vi "Alarms Read.vi"(8 "Error In":errorcluster, 10 "InterfaceData":T1 {"GenEast"."TotalFuel(L)" format="%.2f"; "GenEast"."FuelRate(L/H)" format="%.2f"; "GenEast"."ApparentPower(VA)" format="%.2f"; "GenEast"."BattVoltage(V)" format="%.2f"; "GenEast"."Freq(Hz)" format="%.2f"; "GenEast"."RunHours(hr)" format="%.2f"; "GenEast"."PowerFactor" format="%.2f"; "GenEast"."ReactivePower(VAR)" format="%.2f"; "GenEast"."ActivePower(W)" format="%.2f"; "GenWest"."TotalFuel(L)" format="%.2f"; "GenWest"."FuelRate(L/H)" format="%.2f"; "GenWest"."ApparentPower(VA)" format="%.2f"; "GenWest"."BattVoltage(V)" format="%.2f"; "GenWest"."Freq(Hz)" format="%.2f"; "GenWest"."RunHours(hr)" format="%.2f"; "GenWest"."PowerFactor" format="%.2f"; "GenWest"."ReactivePower(VAR)" format="%.2f"; "GenWest"."ActivePower(W)" format="%.2f"; "Converter Alarms 2" format="%016b"; "Converter Faults 2" format="%016b"; "Controller Faults" format="%016b"; "System Status" format="%016b"; "Converter Alarms 1" format="%016b"; "Converter Faults 1" format="%016b"; "Solar Faults" format="%016b"; "ES Rack 10 Alarms" format="%016b"; "ES Rack 9 Alarms" format="%016b"; "ES Rack 8 Alarms" format="%016b"; "ES Rack 7 Alarms" format="%016b"; "ES Rack 6 Alarms" format="%016b"; "ES Rack 5 Alarms" format="%016b"; "ES Rack 4 Alarms" format="%016b"; "ES Rack 3 Alarms" format="%016b"; "ES Rack 2 Alarms" format="%016b"; "ES Rack 1 Alarms" format="%016b"; "ES System Alarms" format="%016b"; "System Faults" format="%016b"; "ES Rack 10 Faults" format="%016b"; "ES Rack 9 Faults" format="%016b"; "ES Rack 8 Faults" format="%016b"; "ES Rack 7  Faults" format="%016b"; "ES Rack 6 Faults" format="%016b"; "ES Rack 5 Faults" format="%016b"; "ES Rack 4 Faults" format="%016b"; "ES Rack 3 Faults" format="%016b"; "ES Rack 2 Faults" format="%016b"; "ES Rack 1 Faults" format="%016b"; "ES System Faults" format="%016b"}, 11 "Alarms Data In":T3) -> (0 "Error Out":errorcluster, 3 "Alarms Data Out":T3)   [LabVIEW 2014]
uses:
  Controls/Alarms Data.ctl
  Controls/Interface Data.ctl
  Controls/Gen Data.ctl
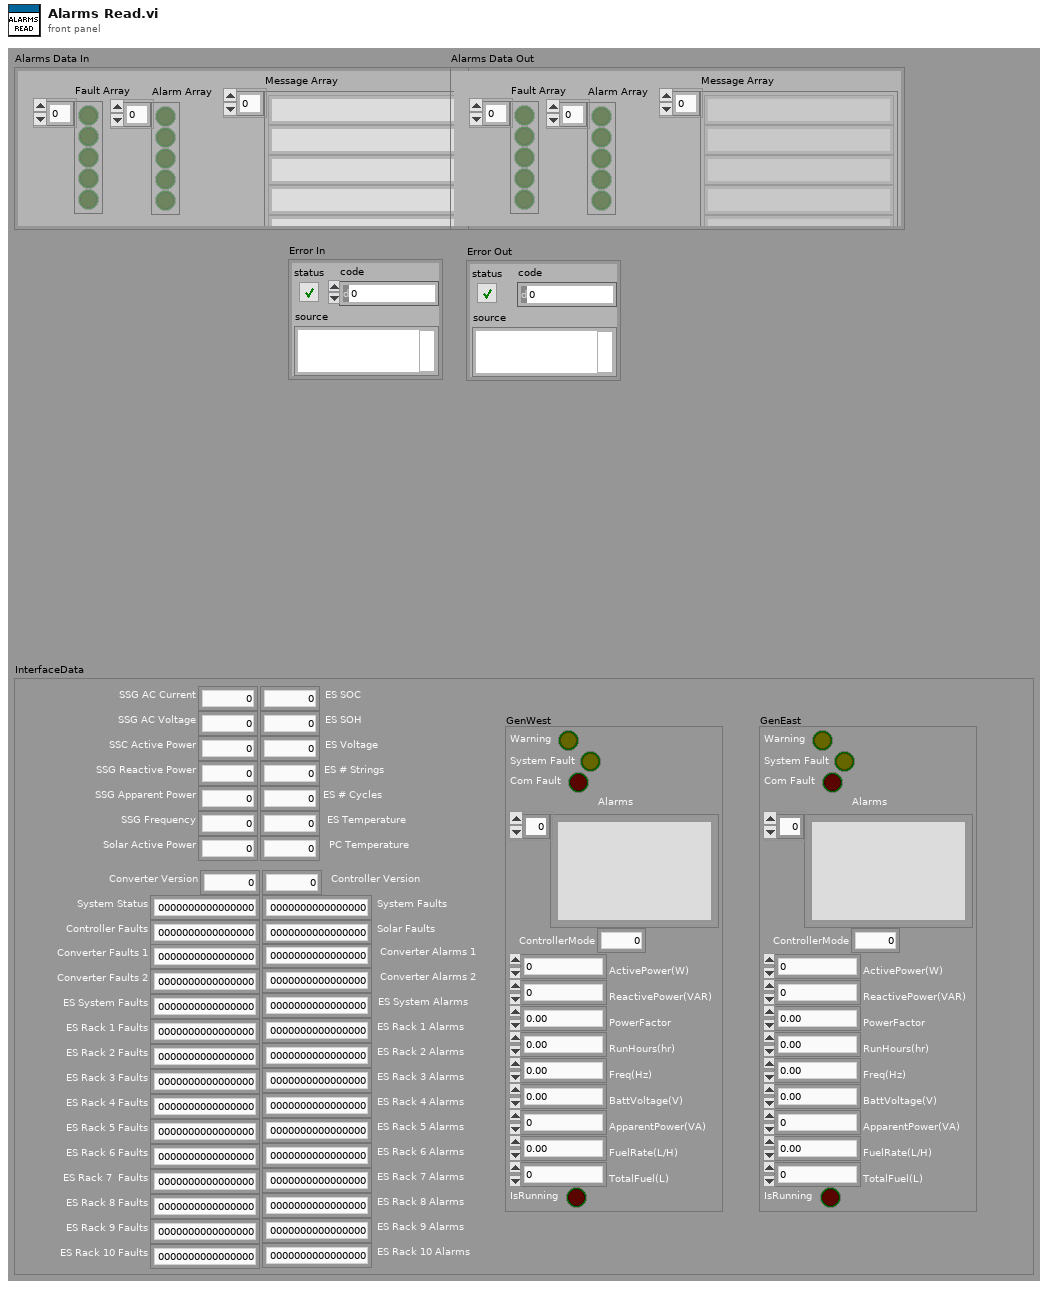
[diagram p1: front panel]
types:
  T1 = typedef "Interface Data.ctl" = cluster{"SSG AC Current":i16, "SSG AC Voltage":i16, "SSC Active Power":i16, "SSG Reactive Power":i16, "SSG Apparent Power":i16, "SSG Frequency":i16, "ES SOC":i16, "ES SOH":i16, "ES Voltage":i16, "ES # Strings":i16, "ES # Cycles":i16, "ES Temperature":i16, "PC Temperature":i16, "Solar Active Power":i16, "Converter Version":i16, "Controller Version":i16, "System Status":i16, "System Faults":i16, "Controller Faults":i16, "ES System Faults":i16, "ES System Alarms":i16, "Converter Faults 1":i16, "Converter Faults 2":i16, "Converter Alarms 1":i16, "Converter Alarms 2":i16, "Solar Faults":i16, "ES Rack 1 Faults":i16, "ES Rack 2 Faults":i16, "ES Rack 3 Faults":i16, "ES Rack 4 Faults":i16, "ES Rack 5 Faults":i16, "ES Rack 6 Faults":i16, "ES Rack 7  Faults":i16, "ES Rack 8 Faults":i16, "ES Rack 9 Faults":i16, "ES Rack 10 Faults":i16, "ES Rack 1 Alarms":i16, "ES Rack 2 Alarms":i16, "ES Rack 3 Alarms":i16, "ES Rack 4 Alarms":i16, "ES Rack 5 Alarms":i16, "ES Rack 6 Alarms":i16, "ES Rack 7 Alarms":i16, "ES Rack 8 Alarms":i16, "ES Rack 9 Alarms":i16, "ES Rack 10 Alarms":i16, "GenWest":T2, "GenEast":T2}
  T2 = typedef "Gen Data.ctl" = cluster{"Warning":bool, "System Fault":bool, "Com Fault":bool, "Alarms":string[], "ControllerMode":u16, "ActivePower(W)":i32, "ReactivePower(VAR)":i32, "PowerFactor":dbl, "RunHours(hr)":dbl, "Freq(Hz)":dbl, "BattVoltage(V)":dbl, "ApparentPower(VA)":i32, "FuelRate(L/H)":dbl, "TotalFuel(L)":u32, "IsRunning":bool}
  T3 = typedef "Alarms Data.ctl" = cluster{"Message Array":string[], "Fault Array":bool[], "Alarm Array":bool[]}
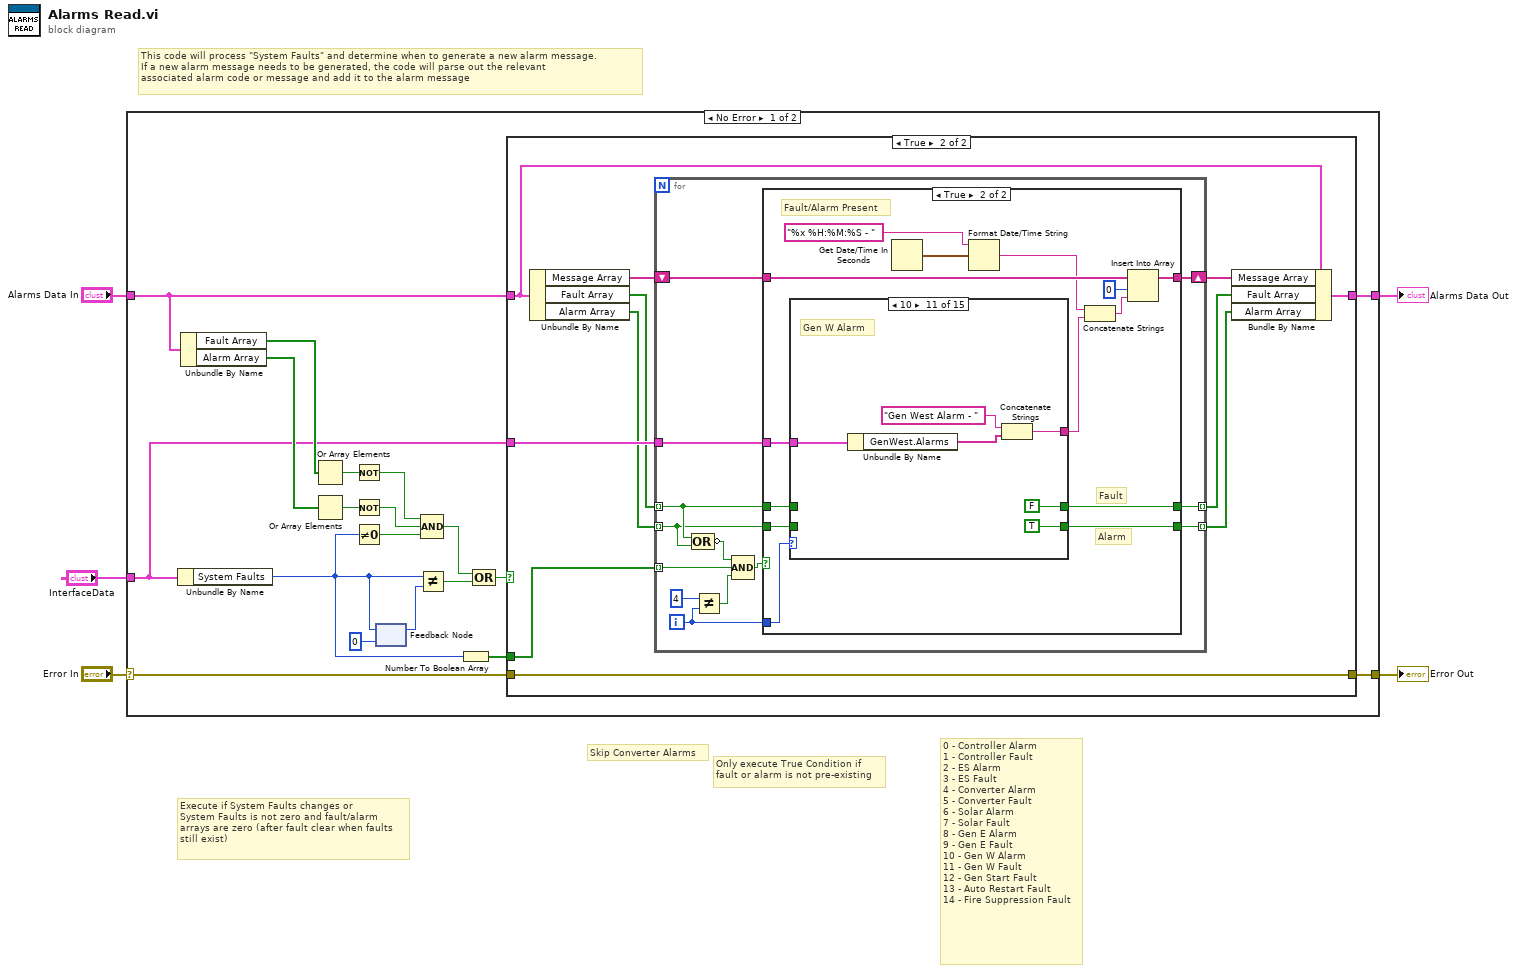
[diagram p0: block diagram]
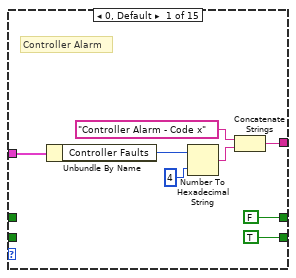
[diagram p4: hidden frame]
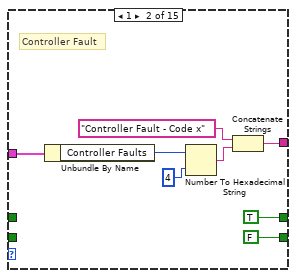
[diagram p5: hidden frame]
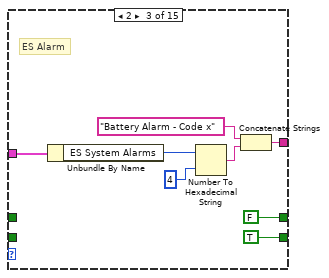
[diagram p6: hidden frame]
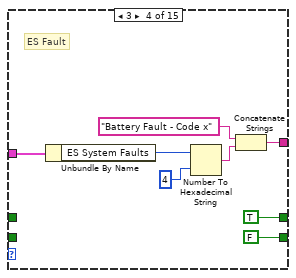
[diagram p7: hidden frame]
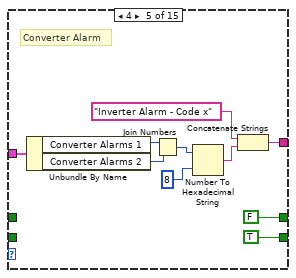
[diagram p8: hidden frame]
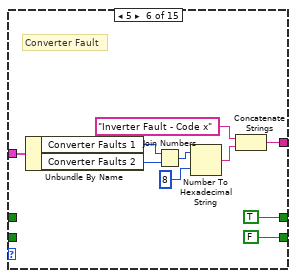
[diagram p9: hidden frame]
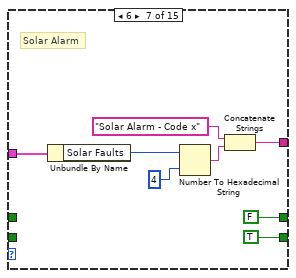
[diagram p10: hidden frame]
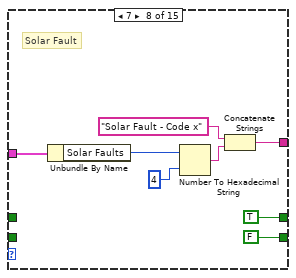
[diagram p11: hidden frame]
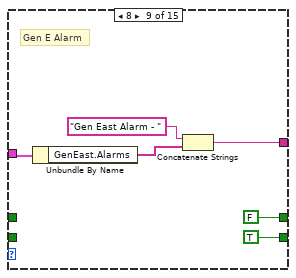
[diagram p12: hidden frame]
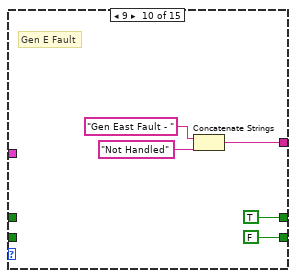
[diagram p13: hidden frame]
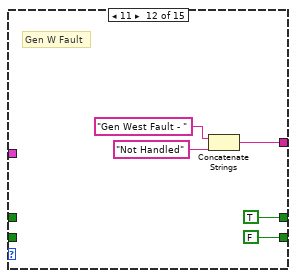
[diagram p14: hidden frame]
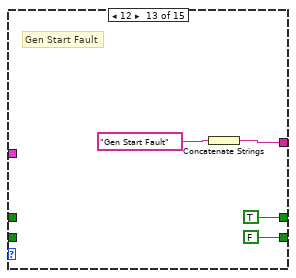
[diagram p15: hidden frame]
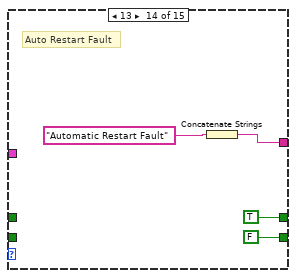
[diagram p16: hidden frame]
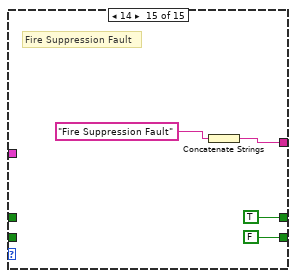
[diagram p17: hidden frame]
diagram:
  # "Skip Converter Alarms"
  # "This code will process \"System Faults\" and determine when to generate a new alarm message.  \nIf a new alarm message needs to be generated, the code will parse out the relevant \nassociated alarm code or message and add it to the alarm message"
  # "Execute if System Faults changes or \nSystem Faults is not zero and fault/alarm\narrays are zero (after fault clear when faults \nstill exist)"
  # "Only execute True Condition if \nfault or alarm is not pre-existing"
  # "0 - Controller Alarm\n1 - Controller Fault\n2 - ES Alarm\n3 - ES Fault\n4 - Converter Alarm\n5 - Converter Fault\n6 - Solar Alarm\n7 - Solar Fault\n8 - Gen E Alarm\n9 - Gen E Fault\n10 - Gen W Alarm\n11 - Gen W Fault\n12 - Gen Start Fault\n13 - Auto Restart Fault\n14 - Fire Suppression Fault"
  n1 = case shown="No Error" "Error In" {
    selector: "Error In" -> [w24 w171]
    tunnel: [w23 w171] -> w4
    tunnel: "Alarms Data In" -> [w17 w170]
    tunnel: [w20 w170] -> w2
    tunnel: "InterfaceData" -> [w9 _]
    frame No Error {
      n2 = Unbundle By Name(w9) -> ("System Faults"=w6:i16)
      n3 = Unbundle By Name(w17) -> ("Fault Array"=w15:bool[], "Alarm Array"=w14:bool[])
      n4 = Or Array Elements(Boolean array=w15) -> (logical OR=w8:bool)
      n5 = Or Array Elements(Boolean array=w14) -> (logical OR=w7:bool)
      n6 = Not(x=w8) -> (.not. x?=w11:bool)
      n7 = Not(x=w7) -> (.not. x?=w12:bool)
      n8 = Not Equal To 0?(x=w6) -> (x != 0?=w16:bool)
      n9 = feedback-in #1(w6) -> ()
      n10 = feedback #1(i16 0 ("System Faults (30052)")) -> (w21:i16)
      n11 = Not Equal?(x=w6, y=w21) -> (x != y?=w19:bool)
      n12 = Compound Arithmetic op=AND(w11, w12, w16) -> (w13:bool)
      n13 = Number To Boolean Array(number=w6) -> (Boolean array=w10:bool[])
      n14 = Compound Arithmetic op=OR(w13, w19) -> (w18:bool)
      n15 = case shown="True" w18 {
        tunnel: w24 -> [w25 w37]
        tunnel: [w25 w37] -> w23
        tunnel: w17 -> [w26 w29]
        tunnel: [w26 w36] -> w20
        tunnel: w10 -> [_ w35]
        tunnel: w9 -> [_ w34]
        frame False {
        }
        frame True {
          n16 = Unbundle By Name(w29) -> ("Message Array"=w30:string[], "Fault Array"=w33:bool[], "Alarm Array"=w32:bool[])
          n17 = for {
            tunnel: w35 -> [w45] mode=indexing
            tunnel: w34 -> [w50]
            tunnel: w33 -> [w43] mode=indexing
            tunnel: w32 -> [w42] mode=indexing
            shift-right: [w48] -> w31
            shift-left: w30 -> [w49]
            tunnel: [w47] -> w28 mode=indexing
            tunnel: [w46] -> w27 mode=indexing
            i -> [w40]
            n18 = Compound Arithmetic op=OR(w43, w42) -> (invert w41:bool)
            n19 = Not Equal?(x=4, y=w40) -> (x != y?=w39:bool)
            n20 = Compound Arithmetic op=AND(w41, w45, w39) -> (w44:bool)
            n21 = case shown="True" w44 {
              tunnel: w40 -> [_ w67]
              tunnel: w50 -> [_ w66]
              tunnel: w49 -> [w53 w65]
              tunnel: [w53 w63] -> w48
              tunnel: w43 -> [w52 w62]
              tunnel: [w52 w59] -> w47
              tunnel: w42 -> [w51 w61]
              tunnel: [w51 w60] -> w46
              frame False {
                # "No Fault/Alarm Present"
              }
              frame True {
                # "Fault/Alarm Present"
                # "Alarm"
                # "Fault"
                n22 = case shown="10" w67 {
                  tunnel: w66 -> [w70 w81 w88 w93 w104 w114 w121 w129 w137 _ w148 _ _ _ _]
                  tunnel: [w69 w80 w84 w92 w103 w113 w120 w128 w138 w143 w149 w154 w158 w162 w166] -> w55
                  tunnel: w62 -> [_ _ _ _ _ _ _ _ _ _ _ _ _ _ _]
                  tunnel: w61 -> [_ _ _ _ _ _ _ _ _ _ _ _ _ _ _]
                  tunnel: [TRUE FALSE TRUE FALSE TRUE FALSE TRUE FALSE TRUE FALSE TRUE FALSE FALSE FALSE FALSE] -> w60
                  tunnel: [FALSE TRUE FALSE TRUE FALSE TRUE FALSE TRUE FALSE TRUE FALSE TRUE TRUE TRUE TRUE] -> w59
                  frame 0, Default {
                    # "Controller Alarm"
                    n23 = Unbundle By Name(w70) -> ("Controller Faults"=w73:i16)
                    n24 = Number To Hexadecimal String(1:i16 4 ("width (-)"), 2:w73) -> (0:w71:string)
                    n25 = Concatenate Strings("Controller Alarm - Code x" ("string"), w71) -> (w69:string)
                  }
                  frame 1 {
                    # "Controller Fault"
                    n26 = Unbundle By Name(w81) -> ("Controller Faults"=w78:i16)
                    n27 = Number To Hexadecimal String(1:i16 4 ("width (-)"), 2:w78) -> (0:w76:string)
                    n28 = Concatenate Strings("Controller Fault - Code x" ("Message Array"), w76) -> (w80:string)
                  }
                  frame 2 {
                    # "ES Alarm"
                    n29 = Unbundle By Name(w88) -> ("ES System Alarms"=w86:i16)
                    n30 = Number To Hexadecimal String(1:i16 4 ("width (-)"), 2:w86) -> (0:w85:string)
                    n31 = Concatenate Strings("Battery Alarm - Code x" ("Message Array"), w85) -> (w84:string)
                  }
                  frame 3 {
                    # "ES Fault"
                    n32 = Unbundle By Name(w93) -> ("ES System Faults"=w95:i16)
                    n33 = Number To Hexadecimal String(1:i16 4 ("width (-)"), 2:w95) -> (0:w94:string)
                    n34 = Concatenate Strings("Battery Fault - Code x" ("Message Array"), w94) -> (w92:string)
                  }
                  frame 4 {
                    # "Converter Alarm"
                    n35 = Unbundle By Name(w104) -> ("Converter Alarms 1"=w102:i16, "Converter Alarms 2"=w101:i16)
                    n36 = Join Numbers(hi=w102, lo=w101) -> ((hi.lo)=w100:u32)
                    n37 = Number To Hexadecimal String(1:i16 8 ("width (-)"), 2:w100) -> (0:w105:string)
                    n38 = Concatenate Strings("Inverter Alarm - Code x" ("Message Array"), w105) -> (w103:string)
                  }
                  frame 5 {
                    # "Converter Fault"
                    n39 = Unbundle By Name(w114) -> ("Converter Faults 1"=w112:i16, "Converter Faults 2"=w111:i16)
                    n40 = Join Numbers(hi=w112, lo=w111) -> ((hi.lo)=w110:u32)
                    n41 = Number To Hexadecimal String(1:i16 8 ("width (-)"), 2:w110) -> (0:w115:string)
                    n42 = Concatenate Strings("Inverter Fault - Code x" ("Message Array"), w115) -> (w113:string)
                  }
                  frame 6 {
                    # "Solar Alarm"
                    n43 = Unbundle By Name(w121) -> ("Solar Faults"=w123:i16)
                    n44 = Number To Hexadecimal String(1:i16 4 ("width (-)"), 2:w123) -> (0:w122:string)
                    n45 = Concatenate Strings("Solar Alarm - Code x" ("Message Array"), w122) -> (w120:string)
                  }
                  frame 7 {
                    # "Solar Fault"
                    n46 = Unbundle By Name(w129) -> ("Solar Faults"=w131:i16)
                    n47 = Number To Hexadecimal String(1:i16 4 ("width (-)"), 2:w131) -> (0:w130:string)
                    n48 = Concatenate Strings("Solar Fault - Code x" ("Message Array"), w130) -> (w128:string)
                  }
                  frame 8 {
                    # "Gen E Alarm"
                    n49 = Unbundle By Name(w137) -> ("GenEast.Alarms"=w136:string[])
                    n50 = Concatenate Strings("Gen East Alarm - " ("Message Array"), w136) -> (w138:string)
                  }
                  frame 9 {
                    # "Gen E Fault"
                    n51 = Concatenate Strings("Gen East Fault - " ("Message Array"), "Not Handled" ("string")) -> (w143:string)
                  }
                  frame 10 {
                    # "Gen W Alarm"
                    n52 = Unbundle By Name(w148) -> ("GenWest.Alarms"=w147:string[])
                    n53 = Concatenate Strings("Gen West Alarm - " ("Message Array"), w147) -> (w149:string)
                  }
                  frame 11 {
                    # "Gen W Fault"
                    n54 = Concatenate Strings("Gen West Fault - " ("Message Array"), "Not Handled" ("string")) -> (w154:string)
                  }
                  frame 12 {
                    # "Gen Start Fault"
                    n55 = Concatenate Strings("Gen Start Fault" ("Message Array")) -> (w158:string)
                  }
                  frame 13 {
                    # "Auto Restart Fault"
                    n56 = Concatenate Strings("Automatic Restart Fault" ("Message Array")) -> (w162:string)
                  }
                  frame 14 {
                    # "Fire Suppression Fault"
                    n57 = Concatenate Strings("Fire Suppression Fault" ("Message Array")) -> (w166:string)
                  }
                }
                n58 = Get Date/Time In Seconds() -> (seconds since 1Jan1904=w57:timestamp)
                n59 = Format Date/Time String(time format string (%c)="%x %H:%M:%S - ", seconds (now)=w57) -> (date/time string=w56:string)  [unwired: 1 in]
                n60 = Concatenate Strings(w56, w55) -> (w64:string)
                n61 = Insert Into Array(array=w65, index=0, new element=w64) -> (w63:string[])
              }
            }
          }
          n62 = Bundle By Name(cluster=w29, "Message Array"=w31, "Fault Array"=w28, "Alarm Array"=w27) -> (w36:T3)
        }
      }
    }
    frame Error {
    }
  }
  "Error Out" <- w4
  "Alarms Data Out" <- w2
